vi "FarFiledCamSetExposure.vi"(3 "曝光时间us":dbl) -> (0 "设置成功":bool, 1 "当前曝光us":dbl)   [LabVIEW 2018]
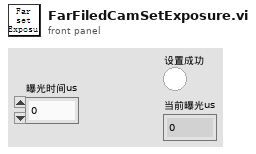
[diagram p1: front panel]
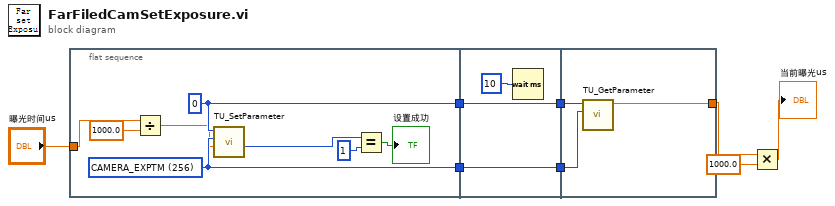
[diagram p0: block diagram]
diagram:
  n1 = flat-sequence {
    tunnel: "曝光时间us" -> [w11]
    tunnel: [w16] -> w7
    tunnel: [w15] -> w5
    tunnel: w7 -> [w19]
    tunnel: [w19] -> w6
    tunnel: w5 -> [w18]
    tunnel: [w18] -> w4
    tunnel: w6 -> [w22]
    tunnel: w4 -> [w21]
    tunnel: [w20] -> w3
    frame #0 {
      w15 = u32 256 items=["CAMERA_EXPTM"=256, "CAMERA_RGAIN"=261, "CAMERA_GGAIN"=266, "CAMERA_BGAIN"=271, "CAMERA_SATURATION"=276, "CAMERA_GAMMA"=281, "CAMERA_CONTRAST"=286, "CAMERA_AUTOWB"=512] ("Parameter")
      w16 = i16 0 ("Camera Index")
      n2 = Divide(x=w11, y=1000.0) -> (x/y=w9:dbl)
      n3 = call <userlib>:"TU_SetParameter.vi"("Value in"=w9, "Parameter"=w15, "Camera Index"=w16) -> ("Return Value"=w14:u32)  [unwired: 4 in]
      n4 = Equal?(x=w14, y=u32 1) -> (x = y?=→"设置成功":bool)
    }
    frame #1 {
      n5 = Wait (ms)(milliseconds to wait=u32 10 ("等待时间（毫秒）")) -> ()  [unwired: 1 out]
    }
    frame #2 {
      n6 = call <userlib>:"TU_GetParameter.vi"("Parameter ID"=w21, "Camera Index"=w22) -> ("Parameter Value"=w20:dbl)  [unwired: 6 in, 3 out]
    }
  }
  n7 = Multiply(x=w3, y=1000.0) -> (x*y=→"当前曝光us":dbl)
